vi "Process.vi"(11 "Actor":refnum<class "Dev View.lvclass">) -> ()   [LabVIEW 2021, in "Dev View.lvclass"]
uses:
  Dev View.lvclass
  Dev View.lvclass/Dev View.ctl
  Re-use Libraries/Minimal Actor Framework/Actors/Base Actor/Actor/Front Panel State.ctl
  Re-use Libraries/Minimal Actor Framework/Actors/Base Actor/Actor/Actor.lvclass
  Re-use Libraries/Minimal Actor Framework/Messaging/Message/Message.lvclass
  Actors/Error Handler/API/Error Handler Actor API.lvclass
  Actors/Main Controller/API/Main Controller Actor API.lvclass
  Actors/Main Controller/Actor/Windows.ctl
  Actors/Main Controller/Actor/Main Controller Actor.lvclass
  Re-use Libraries/Utility/UI/System Button (without mouse hover).ctl
  Re-use Libraries/Utility/Utility.lvlib
panel:
  in  "Actor Debugger":T1
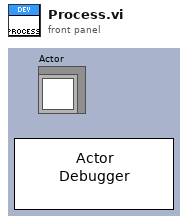
[diagram p1: front panel]
types:
  T1 = typedef "Utility.lvlib/System Button (without mouse hover).ctl" = bool
  T2 = typedef "Actor.lvclass/Front Panel State.ctl" = enum32{"Invalid", "Standard", "Closed", "Hidden", "Minimized", "Maximized"}
  T3 = typedef "Main Controller Actor.lvclass/Windows.ctl" = enum16{"About", "Debugger"}
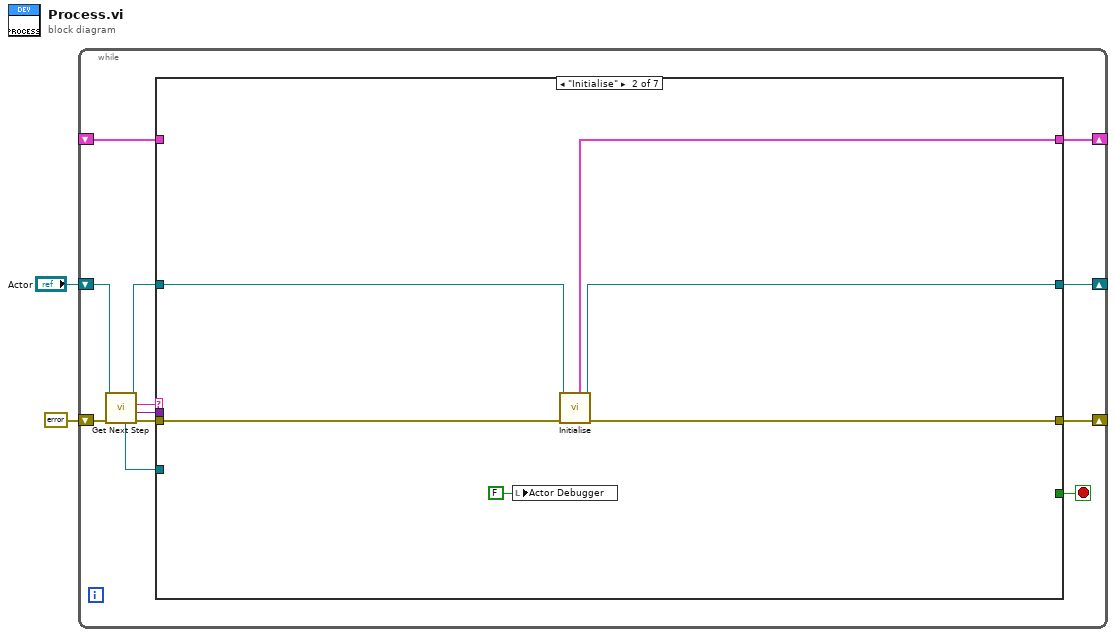
[diagram p0: block diagram]
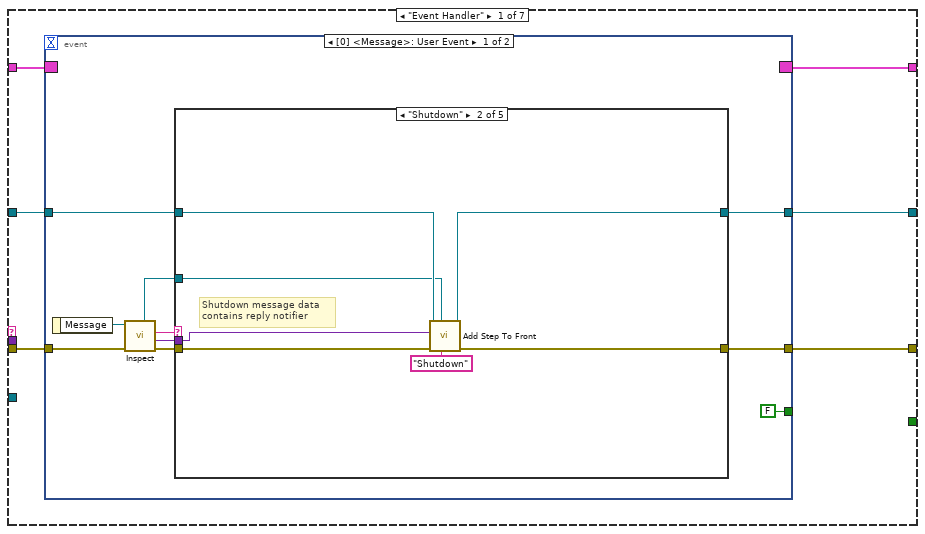
[diagram p2: hidden frame]
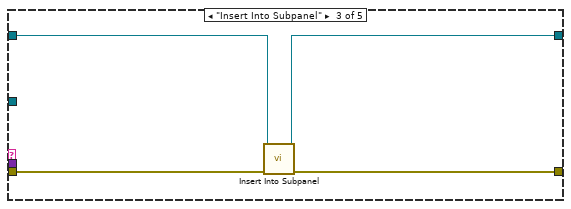
[diagram p4: hidden frame]
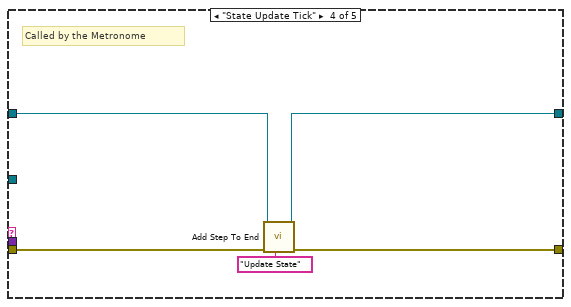
[diagram p5: hidden frame]
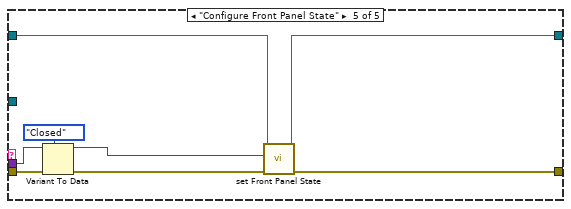
[diagram p6: hidden frame]
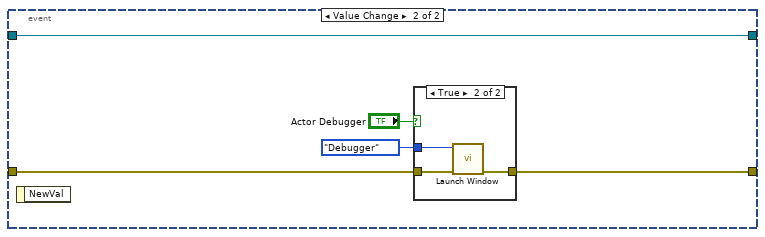
[diagram p7: hidden frame]
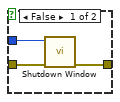
[diagram p8: hidden frame]
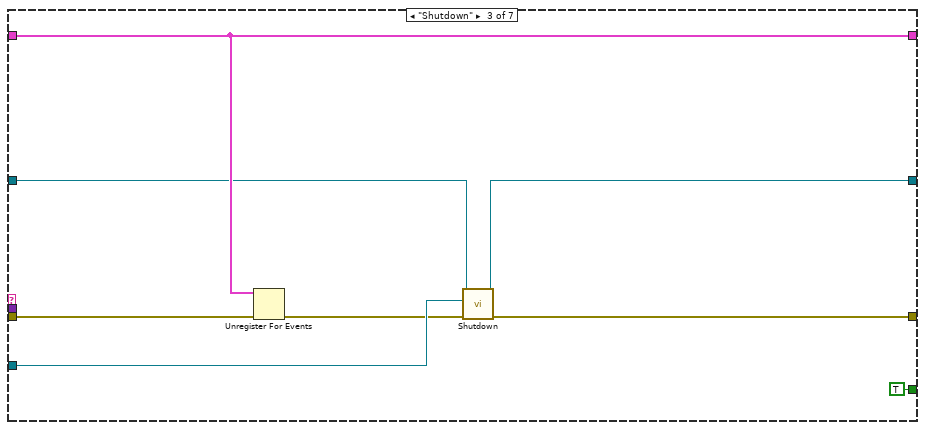
[diagram p9: hidden frame]
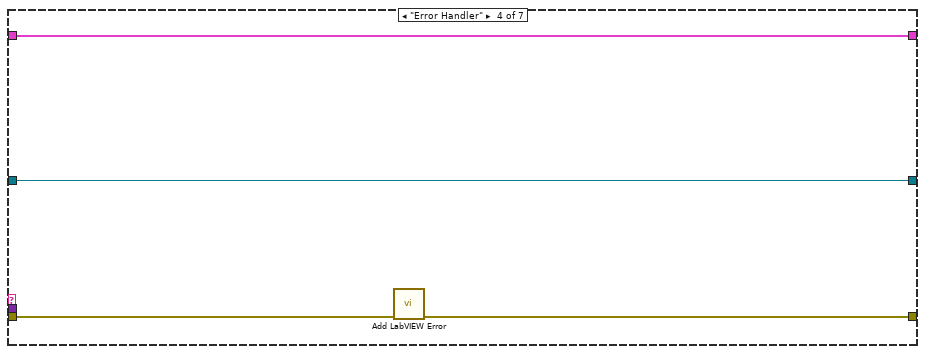
[diagram p10: hidden frame]
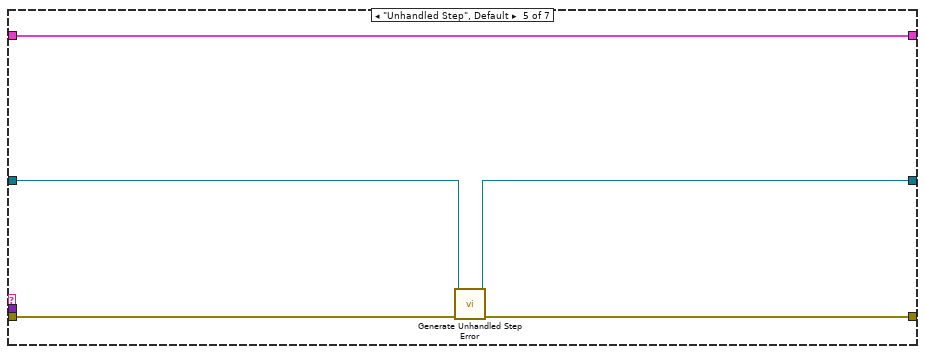
[diagram p11: hidden frame]
diagram:
  n1 = while {
    shift-right: [w5] -> _
    shift-left: "Actor" -> [w13]
    shift-right: [w10] -> _
    shift-left: _ -> [w9]
    shift-right: [w4] -> _
    shift-left: errorcluster {"status"=FALSE, "code"=0, "source"=""} ("error constant") -> [w7]
    stop <- w14 stop-if-true
    n2 = call-dynamic "Get Next Step.vi"("error in (no error)"=w7, "Actor in"=w13) -> ("error out"=w8:errorcluster, "Parameter"=w11:variant, "Step"=w6:string, "Actor out"=w12:refnum<class "Dev View.lvclass">, "Reply Channel"=w3:refnum<notifier>)  [unwired: 5 in]
    n3 = case shown="\"Initialise\"" w6 {
      tunnel: [_ _ TRUE _ _ _ _] -> w14
      tunnel: w12 -> [w20 w70 w74 w82 w89 w92 w94]
      tunnel: [w19 w71 w79 w82 w88 w92 w94] -> w5
      tunnel: w11 -> [_ _ _ _ _ _ _]
      tunnel: [w17 w73 w80 w85 w90 w93 w96] -> w10
      tunnel: w9 -> [w18 _ w80 w85 w90 w93 w96]
      tunnel: w8 -> [w16 w68 w77 w84 w87 w91 w95]
      tunnel: [w15 w72 w75 w83 w86 w91 w95] -> w4
      tunnel: w3 -> [_ _ w78 _ _ _ _]
      frame "Event Handler" {
        n4 = event shown="[0] <Message>: User Event" {
          selector: w18 -> [_ _]
          dyn-events: [_ _] -> w17
          timeout: _ -> [_ _]
          tunnel: w20 -> [w30 w61]
          tunnel: [w29 w61] -> w19
          tunnel: w16 -> [w27 w60]
          tunnel: [w28 w59] -> w15
          tunnel: [FALSE _] -> _
          event User Event {
            n5 = event-data() -> ("Message"=w26:refnum<class "Message.lvclass">)  [unwired: 1 in]
            n6 = call "Inspect.vi"("error in (no error)"=w27, "Message in"=w26) -> ("error out"=w23:errorcluster, "Data"=w24:variant, "Name"=w25:string, "Reply Channel"=w22:refnum<notifier>)  [unwired: 5 in, 1 out]
            n7 = case shown="\"Shutdown\"" w25 {
              tunnel: w30 -> [w32 w39 w43 w48 w56]
              tunnel: [w32 w38 w42 w47 w55] -> w29
              tunnel: w23 -> [w31 w36 w41 w45 w52]
              tunnel: [w31 w35 w40 w44 w54] -> w28
              tunnel: w24 -> [_ w34 _ _ w53]
              tunnel: w22 -> [_ w33 _ _ _]
              frame Default {
              }
              frame "Shutdown" {
                # "Shutdown message data contains reply notifier"
                n8 = call-dynamic "Add Step To Front.vi"("Step Name"="Shutdown", "Reply Channel"=w33, "error in (no error)"=w36, "Parameter"=w34, "Actor in"=w39) -> ("error out"=w35:errorcluster, "Actor out"=w38:refnum<class "Dev View.lvclass">)  [unwired: 5 in]
              }
              frame "Insert Into Subpanel" {
                n9 = call-dynamic "Insert Into Subpanel.vi"("error in (no error)"=w41, "Actor in"=w43) -> ("error out"=w40:errorcluster, "Actor out"=w42:refnum<class "Dev View.lvclass">)  [unwired: 8 in]
              }
              frame "State Update Tick" {
                # "Called by the Metronome"
                n10 = call-dynamic "Add Step To End.vi"("Step Name"="Update State", "error in (no error)"=w45, "Actor in"=w48) -> ("error out"=w44:errorcluster, "Actor out"=w47:refnum<class "Dev View.lvclass">)  [unwired: 7 in]
              }
              frame "Configure Front Panel State" {
                n11 = Variant To Data(error in=w52, type=Front_Panel_State."Closed" ("Front Panel State"), Variant=w53) -> (data=w49:T2, error out=w51:errorcluster)
                n12 = call-dynamic "set Front Panel State.vi"("error in (no error)"=w51, "Front Panel State"=w49, "Actor in"=w56) -> ("error out"=w54:errorcluster, "Actor out"=w55:refnum<class "Dev View.lvclass">)  [unwired: 7 in]
              }
            }
          }
          event Value Change {
            n13 = event-data() -> ()  [unwired: 1 in, 1 out]
            n14 = case shown="True" "Actor Debugger" {
              tunnel: w60 -> [w64 w67]
              tunnel: [w62 w66] -> w59
              tunnel: Windows."Debugger" ("Window") -> [w63 w65]
              frame False {
                n15 = call "Shutdown Window.vi"("error in (no error)"=w64, "Window"=w63) -> ("error out"=w62:errorcluster)  [unwired: 9 in]
              }
              frame True {
                n16 = call "Launch Window.vi"("error in (no error)"=w67, "Window"=w65) -> ("error out"=w66:errorcluster)  [unwired: 9 in]
              }
            }
          }
        }
      }
      frame "Initialise" {
        n17 = local write "Actor Debugger"(FALSE ("Show Actor Debugger")) -> ()
        n18 = call "Initialise.vi"("error in (no error)"=w68, "Actor in"=w70) -> ("error out"=w72:errorcluster, "Actor out"=w71:refnum<class "Dev View.lvclass">, "Observers"=w73:cluster{"Actor":refnum<event-registration>})  [unwired: 7 in]
      }
      frame "Shutdown" {
        n19 = Unregister For Events(event registration refnum=w80, error in=w77) -> (error out=w76:errorcluster)
        n20 = call-dynamic "Shutdown.vi"("error in (no error)"=w76, "Reply Channel"=w78, "Dev View in"=w74) -> ("error out"=w75:errorcluster, "Dev View out"=w79:refnum<class "Dev View.lvclass">)  [unwired: 7 in]
      }
      frame "Error Handler" {
        n21 = call "Add LabVIEW Error.vi"("error in (no error)"=w84) -> ("error out"=w83:errorcluster)  [unwired: 10 in]
      }
      frame "Unhandled Step", Default {
        n22 = call-dynamic "Generate Unhandled Step Error.vi"("error in (no error)"=w87, "Actor in"=w89) -> ("error out"=w86:errorcluster, "Actor out"=w88:refnum<class "Dev View.lvclass">)  [unwired: 8 in]
      }
      frame "-----------------------" {
        # "Separator"
      }
      frame "Update State" {
      }
    }
  }
